vi "Build_Array_RGB.vi"(8 "error in (no error)":errorcluster caption="entrée d'erreur (pas d'erreur)", 11 "Load_SampleImages.lvclass":refnum<class "Load_SampleImages.lvclass">) -> (0 "error out":errorcluster caption="sortie d'erreur", 2 "Image (RGB)":cluster{"Tableau":string[][]}[](array[cluster]), 3 "Load_SampleImages.lvclass":refnum<class "Load_SampleImages.lvclass">)   [LabVIEW 2020, in "Load_SampleImages.lvclass"]
uses:
  Load_SampleImages.lvclass
  Load_SampleImages.lvclass/Load_SampleImages.ctl
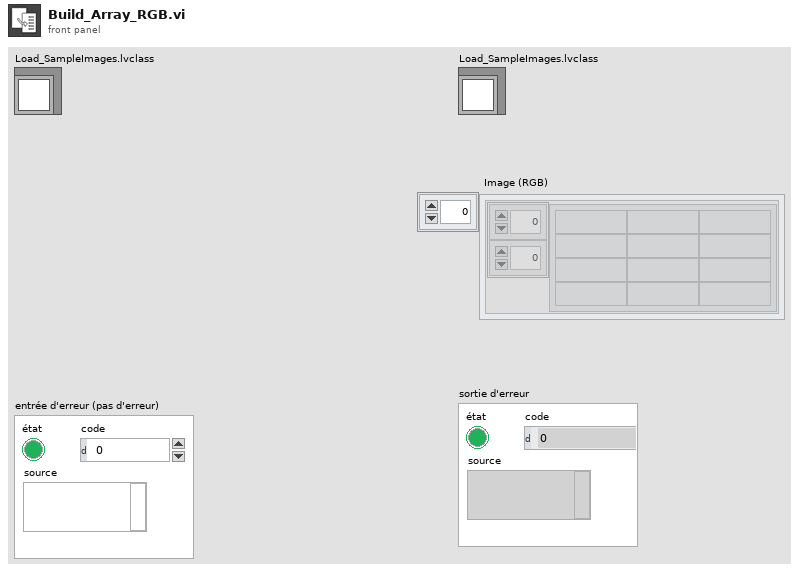
[diagram p1: front panel]
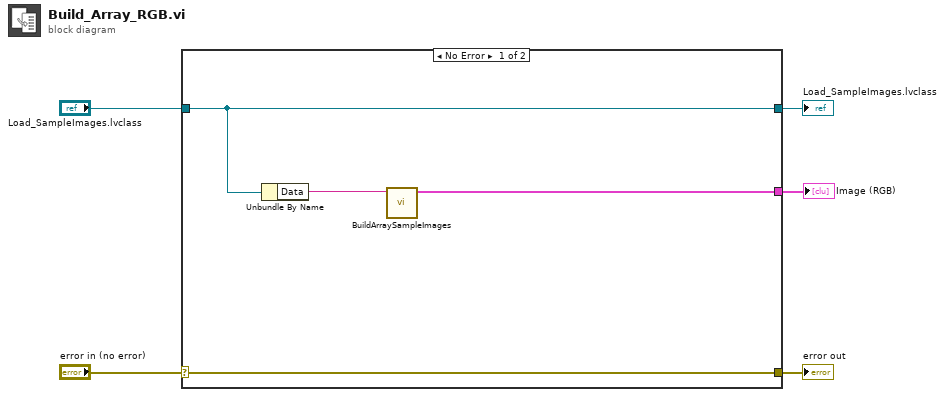
[diagram p0: block diagram]
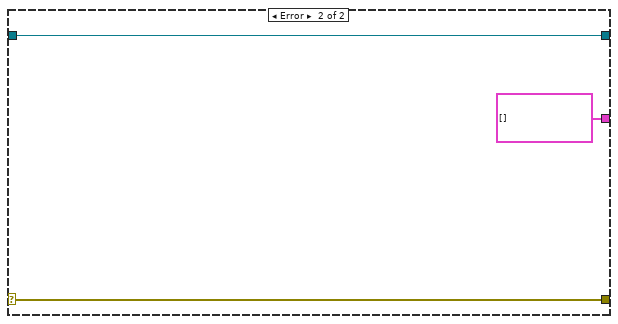
[diagram p2: hidden frame]
diagram:
  n1 = case shown="No Error" "error in (no error)" {
    selector: "error in (no error)" -> [w8 w12]
    tunnel: [w8 w12] -> w4
    tunnel: [w9 w11] -> w2
    tunnel: "Load_SampleImages.lvclass" -> [w9 w11]
    tunnel: [w6 cluster{"Tableau":string[][]}[] [] ("3DArray")] -> w1
    frame No Error {
      n2 = Unbundle By Name(w9) -> ("Data"=w7:string)
      n3 = call "BuildArraySampleImages.vi"("chaîne"=w7) -> ("3DArray"=w6:cluster{"Tableau":string[][]}[])  [unwired: 10 in]
    }
    frame Error {
    }
  }
  "error out" <- w4
  "Load_SampleImages.lvclass" <- w2
  "Image (RGB)" <- w1
